vi "Event Is Refnum.vi"(10 "Event Self":map{string, refnum<data-value>}(c390)) -> (2 "Error":errorcluster)   [LabVIEW 2021, in "jettl.lvlib" / "jettl Queue Actor.lvlib" / "jettl Queue Actor.lvclass"]
uses:
  jettl Queue Actor.lvclass
  Actor/Msg/Msg.lvclass
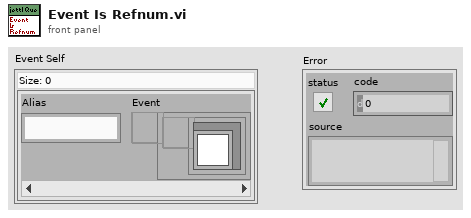
[diagram p1: front panel]
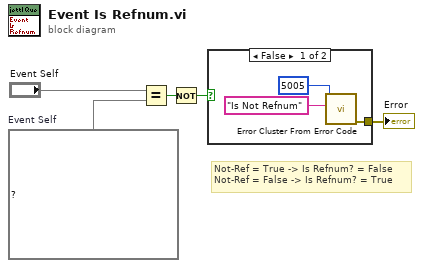
[diagram p0: block diagram]
diagram:
  w1 = map{string, refnum<data-value>} {}  # Event Self
  # "Not-Ref = True -> Is Refnum? = False\nNot-Ref = False -> Is Refnum? = True"
  n1 = Equal?(x="Event Self", y=w1) -> (x = y?=w5:bool)
  n2 = Not(x=w5) -> (.not. x?=w4:bool)
  n3 = case shown="False" w4 {
    tunnel: [w8 _] -> w3
    frame False {
      n4 = call <vilib>:"Error Cluster From Error Code.vi"("error message (\"\")"="Is Not Refnum" ("error message (\"\")"), "error code (0)"=5005) -> ("error out"=w8:errorcluster)  [unwired: 7 in]
    }
    frame True {
    }
  }
  "Error" <- w3
